vi "停止判断1.vi"(7 "反转？":bool, 8 "error in (no error)":errorcluster caption="错误输入（无错误）", 9 "反转判断条件1":T1, 10 "传感器数据":dbl[](array[numeric]), 11 "Message Queues":T2 caption="消息队列") -> (0 "error out":errorcluster caption="错误输出")   [LabVIEW 2015, in "Motor Control.lvlib"]
uses:
  Motor Control.lvlib
  support/Message Queue/All Message Queues.ctl
  support/Message Queue/Message Cluster.ctl
  support/Message Queue/Enqueue Message (Single).vi
  support/Message Queue/Message Queue.lvlib
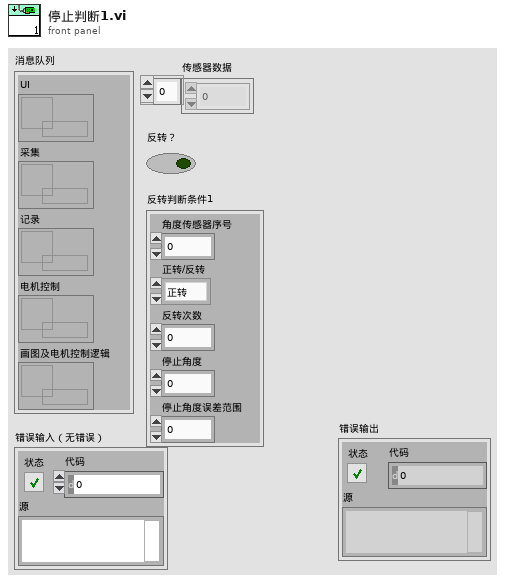
[diagram p1: front panel]
types:
  T1 = typedef "Motor Control.lvlib/停止判断条件1.ctl" = cluster{"角度传感器序号":i32, "正转/反转":enum16{"正转", "反转"}, "反转次数":i32, "停止角度":dbl, "停止角度误差范围":dbl}
  T2 = typedef "Message Queue.lvlib/All Message Queues.ctl" = cluster{"UI":refnum<queue>, "Acquisition":refnum<queue>, "Logging":refnum<queue>, "MotorCtrl":refnum<queue>, "plot logic":refnum<queue>}
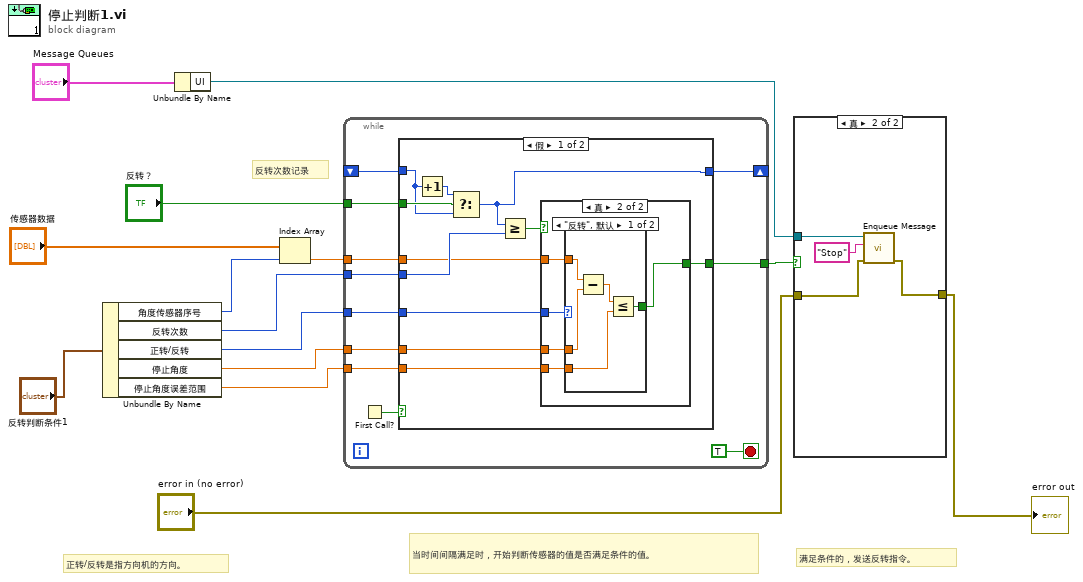
[diagram p0: block diagram]
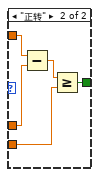
[diagram p4: hidden frame]
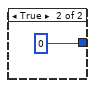
[diagram p5: hidden frame]
diagram:
  # "正转/反转是指方向机的方向。"
  # "满足条件的，发送反转指令。"
  # "当时间间隔满足时，开始判断传感器的值是否满足条件的值。"
  # "反转次数记录"
  n1 = Unbundle By Name("反转判断条件1") -> ("角度传感器序号"=w2:i32, "反转次数"=w11:i32, "正转/反转"=w1:enum16{"正转", "反转"}, "停止角度"=w9:dbl, "停止角度误差范围"=w8:dbl)
  n2 = Unbundle By Name("Message Queues") -> ("UI"=w6:refnum<queue>)
  n3 = Index Array(array="传感器数据", index=w2) -> (element=w10:dbl)
  n4 = while {
    tunnel: w11 -> [w25]
    tunnel: w10 -> [w24]
    tunnel: w9 -> [w23]
    shift-right: [w21] -> _
    shift-left: _ -> [w20]
    tunnel: w8 -> [w19]
    tunnel: [w18] -> w7
    tunnel: "反转？" -> [w16]
    tunnel: w1 -> [w15]
    stop <- TRUE stop-if-true
    n5 = First Call?() -> (First Call?: T/F=w22:bool)
    n6 = case shown="假" w22 {
      tunnel: w25 -> [w32 _]
      tunnel: w24 -> [w30 _]
      tunnel: w23 -> [w28 _]
      tunnel: [w33 0] -> w21
      tunnel: w20 -> [w34 _]
      tunnel: w19 -> [w27 _]
      tunnel: [w26 _] -> w18
      tunnel: w16 -> [w36 _]
      tunnel: w15 -> [w29 _]
      frame False {
        n7 = Increment(x=w34) -> (x+1=w35:i32)
        n8 = Select(t=w35, s=w36, f=w34) -> (s? t:f=w33:i32)
        n9 = Greater Or Equal?(x=w33, y=w32) -> (x >= y?=w31:bool)
        n10 = case shown="真" w31 {
          tunnel: w30 -> [_ w41]
          tunnel: w29 -> [_ w37]
          tunnel: w28 -> [_ w40]
          tunnel: w27 -> [_ w39]
          tunnel: [_ w38] -> w26
          frame False {
          }
          frame True {
            n11 = case shown="\"反转\", 默认" w37 {
              tunnel: w41 -> [w46 w51]
              tunnel: w40 -> [w45 w50]
              tunnel: w39 -> [w43 w48]
              tunnel: [w42 w47] -> w38
              frame "反转", Default {
                n12 = Subtract(x=w46, y=w45) -> (x-y=w44:dbl)
                n13 = Less Or Equal?(x=w44, y=w43) -> (x <= y?=w42:bool)
              }
              frame "正转" {
                n14 = Subtract(x=w51, y=w50) -> (x-y=w49:dbl)
                n15 = Greater Or Equal?(x=w49, y=w48) -> (x >= y?=w47:bool)
              }
            }
          }
        }
      }
      frame True {
      }
    }
  }
  n16 = case shown="真" w7 {
    tunnel: w6 -> [_ w57]
    tunnel: "error in (no error)" -> [w53 w56]
    tunnel: [w53 w55] -> w4
    frame False {
    }
    frame True {
      n17 = call-poly "Enqueue Message.vi"("error in (no error)"=w56, "Message"="Stop", "Message Queue"=w57) -> ("error out"=w55:errorcluster)  [unwired: 7 in, 1 out]
    }
  }
  "error out" <- w4
